vi "merge tx data.vi"(1 "do not merge":bool, 2 "tx data new":cluster{"t":dbl[], "x":dbl[]}, 4 "tx data in":cluster{"t":dbl[], "x":dbl[]}) -> (0 "tx data out":cluster{"t":dbl[], "x":dbl[]})   [LabVIEW 2010]
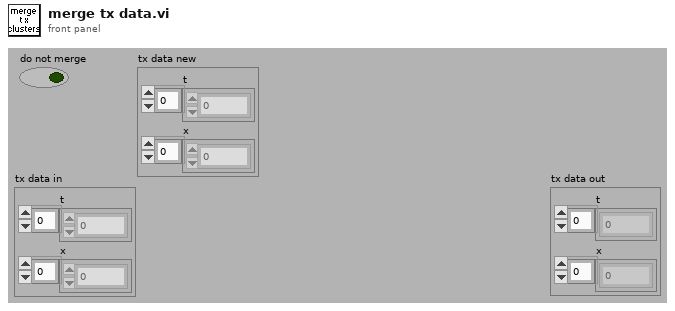
[diagram p1: front panel]
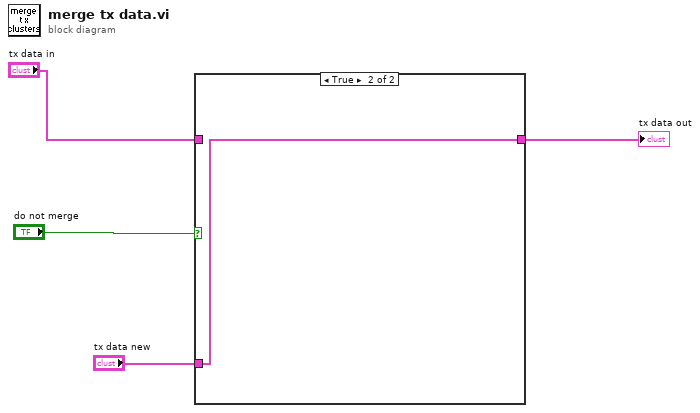
[diagram p0: block diagram]
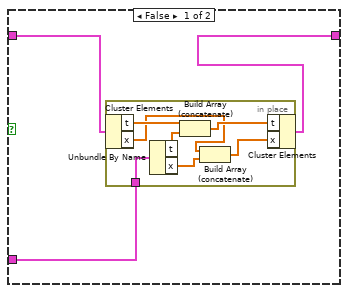
[diagram p2: hidden frame]
diagram:
  n1 = case shown="True" "do not merge" {
    tunnel: "tx data in" -> [w7 _]
    tunnel: [w6 w15] -> w3
    tunnel: "tx data new" -> [w5 w15]
    frame False {
      n2 = in-place {
        in-place-border: w5 -> [w14]
        n3 = in-place-cluster #1(w7) -> ("t"=w13:dbl[], "x"=w9:dbl[])
        n4 = Unbundle By Name(w14) -> ("t"=w12:dbl[], "x"=w10:dbl[])
        n5 = Build Array (concatenate)(w13, w12) -> (w11:dbl[])
        n6 = Build Array (concatenate)(w9, w10) -> (w8:dbl[])
        n7 = in-place-cluster #1("t"=w11, "x"=w8) -> (w6:cluster{"t":dbl[], "x":dbl[]})
      }
    }
    frame True {
    }
  }
  "tx data out" <- w3
